vi "Lockin Proccess.vi"(4 "First call":bool, 6 "CH index":i32, 7 "Harmonics":i32[](array[numeric]), 8 "Error In":errorcluster, 9 "Harmonic":i32=1, 10 "User configuration":T1={"Time constant"=0.0, "Signal channels"=[], "Group"="p", "X channel"="", "Live update"=TRUE, "Phases"=[], "Harmonics"=[]} {"Phases" scale=-180.0..180.0; "Time constant" min=1e-06 max=1.0 scale=1e-06..0.01 scale format="%#_6p"}, 11 "Signal file":path) -> (0 "Error Out":errorcluster, 1 "dt":dbl, 2 "XY Graph":cluster{dbl[], "Y":dbl[]}[](graph), 3 "Signal file out":path, 5 "Signal names":cluster{"Signal Name":string, string[]})   [LabVIEW 2019]
uses:
  LabActor/Post-Processors/Lockin Processor/Lockin Processor Configuration.ctl
  Software Lock-in/Software Lock-in.lvclass
  <vilib>/express/express shared/transition.llb/Dynamic To Waveform Array.vi
  <vilib>/express/express signal manip/GetorSetDDTAttributes/Get DDT Attributes/Get DDT Properties.xnode
panel:
  out "Attempts out":i32
  out "group":string
  out "owner":string
  out "permissions":i16
  out "Deleted channels":string[](array[string])
  out "Waveform Graph 3":dynamicdata(graph)
  out "Waveform Graph 2":dynamicdata(graph)
  out "Waveform Graph":dynamicdata(graph)
  in  "Save output":bool=TRUE
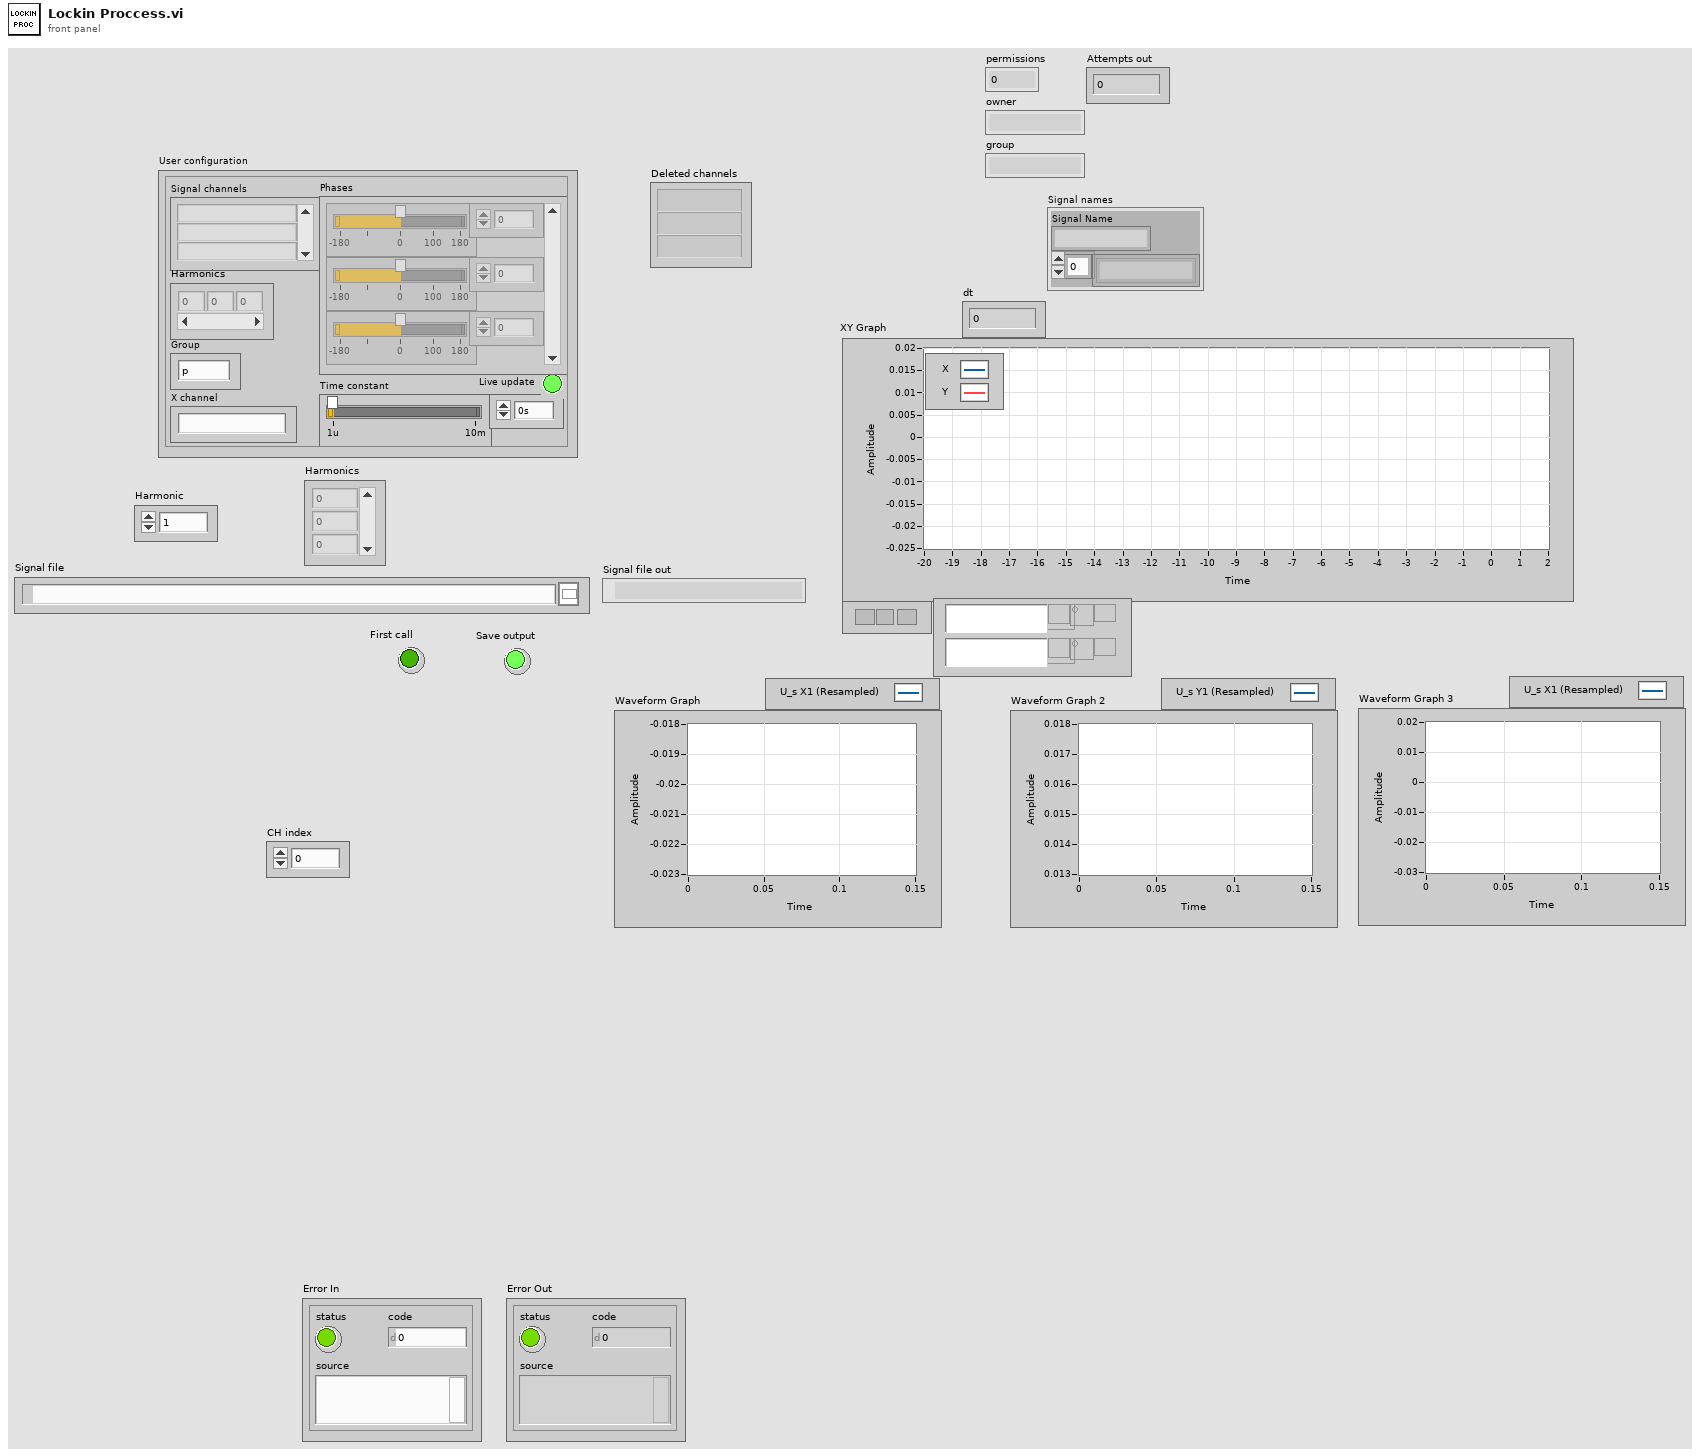
[diagram p1: front panel]
types:
  T1 = typedef "Lockin Processor Configuration.ctl" = cluster{"Time constant":dbl, "Signal channels":string[], "Group":string, "X channel":string, "Live update":bool, "Phases":dbl[], "Harmonics":i32[]}
  T2 = enum16{"open", "open or create", "create or replace", "create", "open (read-only)"}
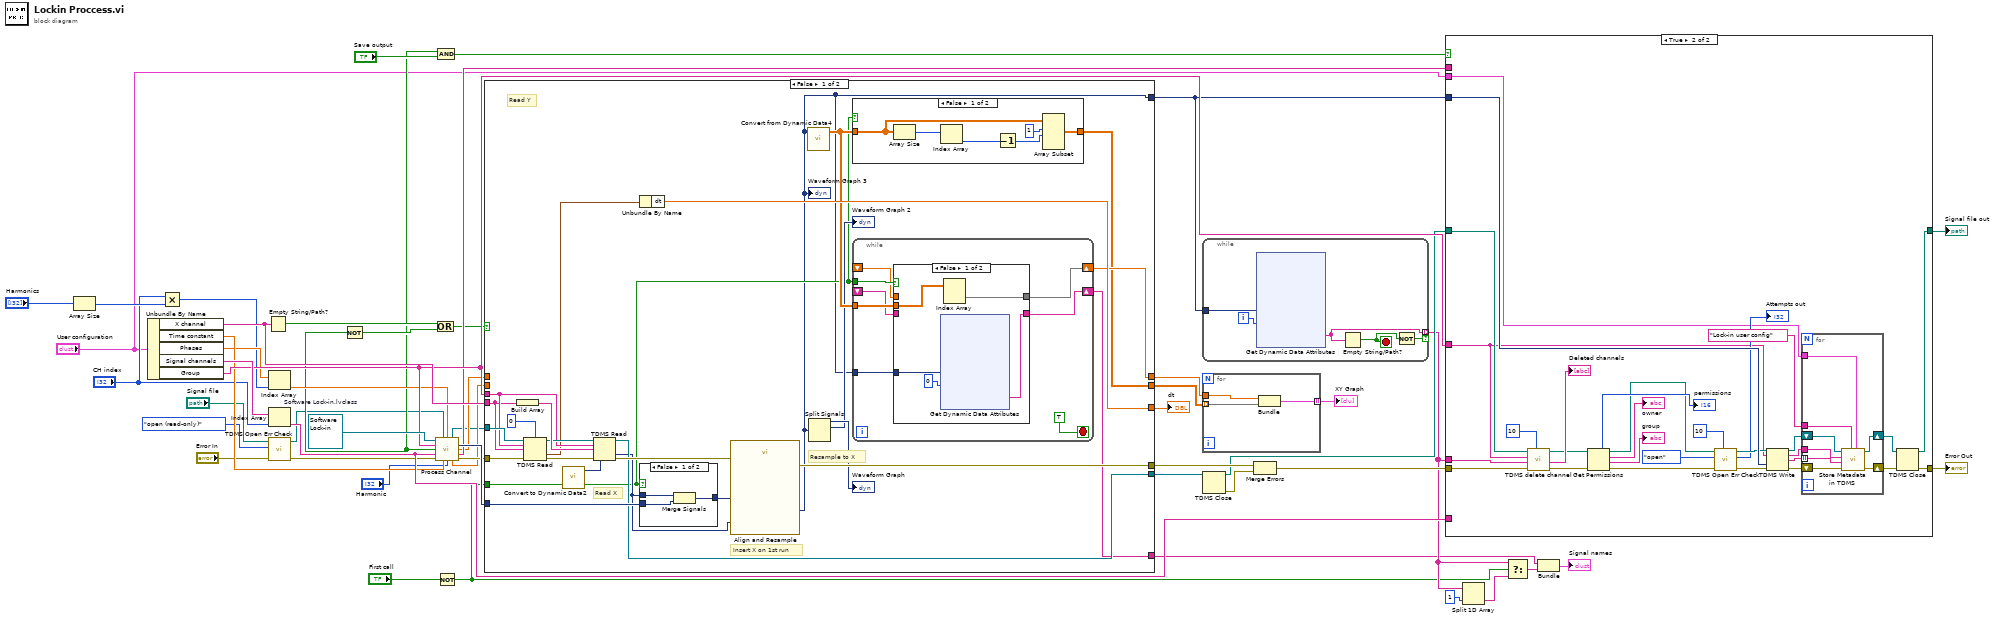
[diagram p0: block diagram]
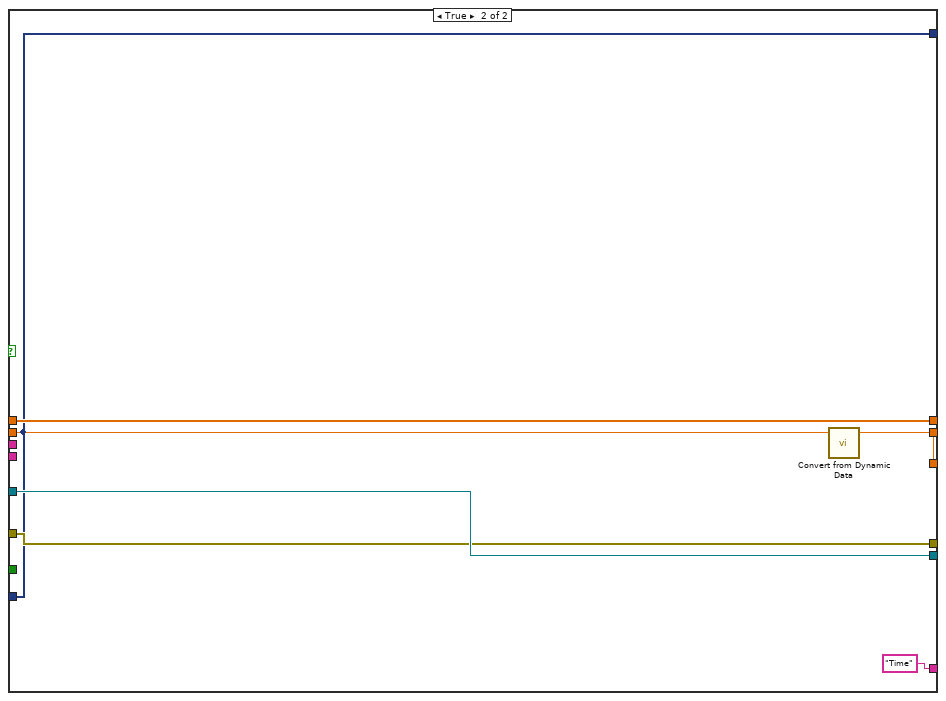
[diagram p5: hidden frame]
diagram:
  w45 = refnum<class "Software Lock-in.lvclass"> refnum  # Software Lock-in.lvclass
  n1 = Array Size(array="Harmonics") -> (size(s)=w13:i32)
  n2 = Unbundle By Name("User configuration") -> ("X channel"=w48:string, "Time constant"=w42:dbl, "Phases"=w21:dbl[], "Signal channels"=w49:string[], "Group"=w44:string)
  n3 = Multiply(x="CH index", y=w13) -> (x*y=w12:i32)
  n4 = Empty String/Path?(string/path=w48) -> (empty?=w26:bool)
  n5 = Index Array(array=w21, index=w12) -> (element=w18:dbl)
  n6 = Index Array(array=w49, index="CH index") -> (element=w43:string)
  n7 = call "TDMS Open Err Check.vi"("Error In"="Error In", "operation (0:open)"=T2."open (read-only)", "File Path Control"="Signal file") -> ("Error Out"=w4:errorcluster, "tdms file out"=w2:refnum<k34>)  [unwired: 6 in, 1 out]
  n8 = call-dynamic "Process Channel.vi"("Software Lock-in in"=w45, "tdms file"=w2, "Phase"=w18, "Group name"=w44, "Channel name"=w43, "error in (no error)"=w4, "Time constant"=w42, "Harmonic"="Harmonic") -> ("tdms file out"=w20:refnum<k34>, "Signal"=w41:dynamicdata, "found"=w7:bool, "Time axis"=w29:dbl[], "Channel names"=w40:string[], "dt"=w32:dbl, "error out"=w37:errorcluster)  [unwired: 1 out]
  n9 = Not(x=w7) -> (.not. x?=w9:bool)
  n10 = Or(x=w26, y=w9) -> (x .or. y?=w10:bool)
  n11 = And(x=w7, y="Save output") -> (x .and. y?=w8:bool)
  n12 = Not(x="First call") -> (.not. x?=w15:bool)
  n13 = case shown="False" w10 {
    tunnel: w41 -> [w76 w114]
    tunnel: w37 -> [w65 w117]
    tunnel: [w74 w117] -> w46
    tunnel: w48 -> [w66 _]
    tunnel: w44 -> [w67 _]
    tunnel: [w53 w114] -> w28
    tunnel: w20 -> [w69 w118]
    tunnel: [w71 w118] -> w39
    tunnel: [w62 w116] -> w33
    tunnel: w32 -> [_ w116]
    tunnel: [w58 w115] -> w31
    tunnel: [w57 w113] -> w30
    tunnel: w29 -> [_ w115]
    tunnel: w15 -> [w54 _]
    tunnel: [w52 "Time"] -> w19
    frame False {
      # "Read Y"
      # "Read X"
      # "Resample to X"
      # "Insert X on 1st run"
      n14 = Build Array(w66) -> (w72:string[])
      n15 = TDMS Read(0:w69, 2:i64 0 ("count (-1: all)"), 5:w67, 7:w66, 11:w65) -> (4:w68:refnum<k34>, 10:w63:waveform(dbl), 15:w64:errorcluster)  [unwired: 3 in, 3 out]
      n16 = call "Convert to Dynamic Data2"() -> ("Dynamic Data Type"=w73:dynamicdata)  [unwired: 4 in]
      n17 = TDMS Read(0:w68, 5:w67, 7:w72, 11:w64, 12:w73) -> (4:w71:refnum<k34>, 10:w60:dynamicdata, 15:w75:errorcluster)  [unwired: 3 in, 3 out]
      n18 = Unbundle By Name(w63) -> ("dt"=w62:dbl)
      n19 = case shown="False" w54 {
        tunnel: w76 -> [w110 w111]
        tunnel: [w109 w111] -> w61
        tunnel: w60 -> [w108 _]
        frame False {
          n20 = Merge Signals(w108, w110) -> (w109:dynamicdata)
        }
        frame True {
        }
      }
      n21 = call "Align and Resample"("Reference Signal"=w60, "error in (no error)"=w75, "Signals"=w61) -> ("error out"=w74:errorcluster, "Resampled Signals"=w53:dynamicdata)  [unwired: 6 in, 1 out]
      "Waveform Graph 3" <- w53
      n22 = call "Convert from Dynamic Data4"("Dynamic Data Type"=w53) -> ("Array"=w59:dbl[][])  [unwired: 3 in]
      n23 = Split Signals(w53) -> (→"Waveform Graph":dynamicdata, →"Waveform Graph 2":dynamicdata)  [unwired: 4 in, 2 out]
      n24 = case shown="False" w54 {
        tunnel: w59 -> [w82 w83]
        tunnel: [w77 w83] -> w57
        frame False {
          n25 = Array Size(array=w82) -> (size(s)=w78:i32[])
          n26 = Index Array(array=w78) -> (element=w79:i32)  [unwired: 1 in]
          n27 = Decrement(x=w79) -> (x-1=w80:i32)
          n28 = Array Subset(array=w82, index (row)=1 ("index"), length (row)=w80) -> (w77:dbl[][])  [unwired: 2 in]
        }
        frame True {
        }
      }
      n29 = while {
        tunnel: w59 -> [w91]
        shift-right: [w90] -> w58
        shift-left: _ -> [w87]
        tunnel: w54 -> [w88]
        shift-right: [w85] -> w52
        shift-left: _ -> [w84]
        tunnel: w53 -> [w86]
        stop <- TRUE stop-if-true
        n30 = case shown="False" w88 {
          tunnel: w91 -> [w96 _]
          tunnel: [w95 w107] -> w90
          tunnel: w87 -> [_ w107]
          tunnel: w86 -> [w94 _]
          tunnel: [w92 w106] -> w85
          tunnel: w84 -> [_ w106]
          frame False {
            n31 = xnode "Get Dynamic Data Attributes"("Signals In"=w94, "Signal Index"=0) -> ("Signal Name"=w92:string)  [unwired: 1 in, 2 out]
            n32 = Index Array(array=w96) -> (element=w95:dbl[])  [unwired: 2 in]
          }
          frame True {
          }
        }
      }
    }
    frame True {
      n33 = call "Convert from Dynamic Data"("Dynamic Data Type"=w114) -> ("Array"=w113:dbl[][])  [unwired: 3 in]
    }
  }
  "dt" <- w33
  n34 = while {
    tunnel: w28 -> [w123]
    tunnel: [w121] -> w24 mode=indexing if=w119
    i -> [w122]
    stop <- w120 stop-if-true
    n35 = xnode "Get Dynamic Data Attributes"("Signals In"=w123, "Signal Index"=w122) -> ("Signal Name"=w121:string)  [unwired: 1 in, 2 out]
    n36 = Empty String/Path?(string/path=w121) -> (empty?=w120:bool)
    n37 = Not(x=w120) -> (.not. x?=w119:bool)
  }
  n38 = for {
    tunnel: w31 -> [w135]
    tunnel: w30 -> [w134] mode=indexing
    tunnel: [w133] -> w36 mode=indexing
    n39 = Bundle("Time axis"=w135, "Array"=w134) -> (w133:cluster{"Time axis":dbl[], "Array":dbl[]})  [unwired: 1 in]
  }
  "XY Graph" <- w36
  n40 = TDMS Close(11:w39) -> (0:w34:errorcluster, 3:w38:path)  [unwired: 1 in]
  n41 = Merge Errors(w46, w34) -> (w35:errorcluster)
  n42 = case shown="True" w8 {
    tunnel: w38 -> [w136 w165]
    tunnel: w35 -> [w137 w164]
    tunnel: [w137 w166] -> w50
    tunnel: w43 -> [_ _]
    tunnel: w44 -> [_ w141]
    tunnel: [w136 w163] -> w47
    tunnel: w28 -> [_ w162]
    tunnel: w40 -> [_ _]
    tunnel: w24 -> [_ w161]
    tunnel: "User configuration" -> [_ w142]
    frame False {
    }
    frame True {
      n43 = call "TDMS delete channel.vi"("Delay"=u32 10, "error in (no error)"=w164, "Channels"=w161, "group name"=w141, "file path"=w165) -> ("error out"=w157:errorcluster, "Deleted channels"=→"Deleted channels":string[], "file path out"=w158:path)  [unwired: 4 in]
      n44 = Get Permissions(8:w157, 11:w158) -> (0:w153:errorcluster, 1:→"group":string, 2:→"owner":string, 3:w152:path, 5:→"permissions":i16)
      n45 = call "TDMS Open Err Check.vi"("Retry attempts"=10, "Error In"=w153, "operation (0:open)"=T2."open", "File Path Control"=w152) -> ("Error Out"=w149:errorcluster, "Attempts out"=→"Attempts out":i32, "tdms file out"=w150:refnum<k34>)  [unwired: 5 in]
      n46 = TDMS Write(0:w150, 5:w141, 9:w162, 11:w149) -> (4:w146:refnum<k34>, 6:w138:string, 8:w140:string[], 15:w144:errorcluster)  [unwired: 2 in]
      n47 = for {
        tunnel: w142 -> [w170]
        shift-right: [w173] -> w145
        shift-left: w146 -> [w174]
        shift-right: [w171] -> w143
        shift-left: w144 -> [w172]
        tunnel: w140 -> [w169] mode=indexing
        tunnel: "Lock-in user config" ("Name") -> [w167]
        tunnel: w138 -> [w168]
        n48 = call "Store Metadata in TDMS.vi"("Value"=w170, "name"=w167, "Error In"=w172, "channel name"=w169, "group name"=w168, "tdms file"=w174) -> ("Error Out"=w171:errorcluster, "tdms file out"=w173:refnum<k34>)  [unwired: 2 in, 2 out]
      }
      n49 = TDMS Close(8:w143, 11:w145) -> (0:w166:errorcluster, 3:w163:path)
    }
  }
  "Error Out" <- w50
  "Signal file out" <- w47
  n50 = Split 1D Array(array=w24, index=1) -> (second subarray=w25:string[])  [unwired: 1 out]
  n51 = Select(t=w24, s=w15, f=w25) -> (s? t:f=w23:string[])
  n52 = Bundle("Signal Name"=w19, w23) -> (→"Signal names":cluster{"Signal Name":string, string[]})  [unwired: 1 in]
